vi "SetMeasureInterval.vi"(7 "SMU":T1, 8 "Error In":errorcluster, 10 "Interval":dbl, 11 "Keithley 2602 In":refnum<visa-resource-name>) -> (0 "Error Out":errorcluster, 3 "Keithley 2602 Out":refnum<visa-resource-name>)   [LabVIEW 2013, in "Keithley-2602.lvlib"]
uses:
  Keithley-2602.lvlib
  Controls/SMU.ctl
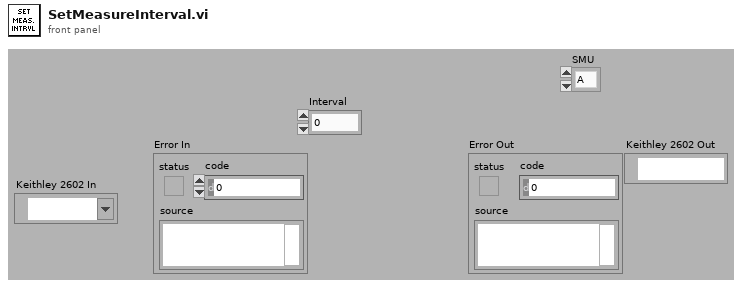
[diagram p1: front panel]
types:
  T1 = typedef "Keithley-2602.lvlib/SMU.ctl" = enum16{"A", "B"}
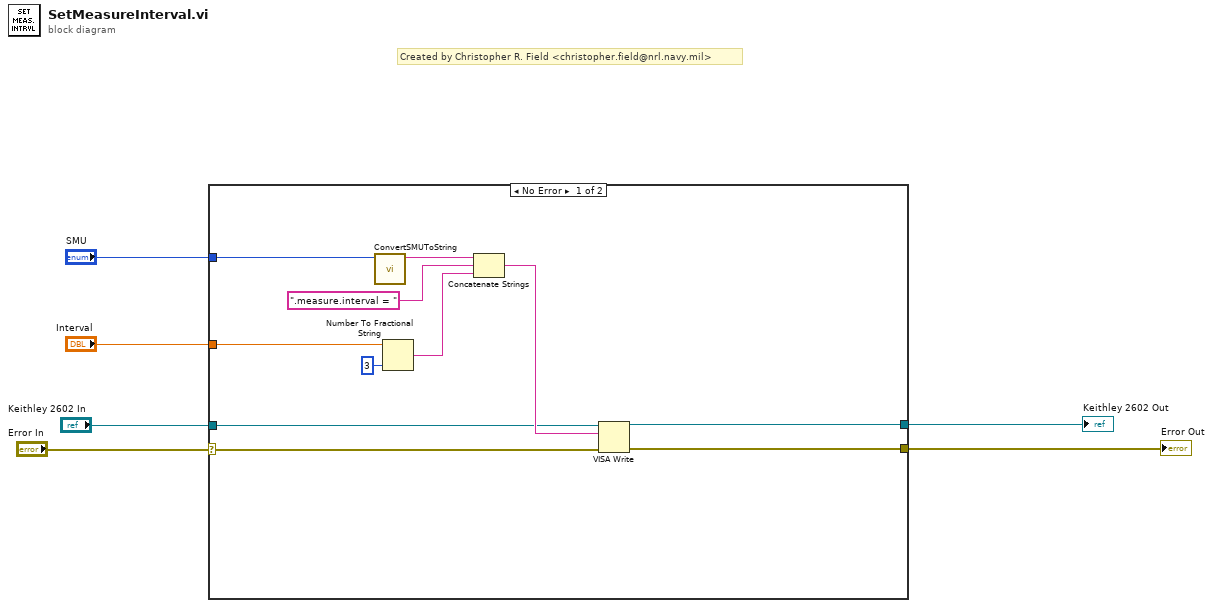
[diagram p0: block diagram]
diagram:
  # "Created by Christopher R. Field <christopher.field@nrl.navy.mil>"
  n1 = case shown="No Error" "Error In" {
    selector: "Error In" -> [w7 w18]
    tunnel: "Keithley 2602 In" -> [w14 w19]
    tunnel: [w13 w18] -> w5
    tunnel: [w12 w19] -> w4
    tunnel: "Interval" -> [w11 _]
    tunnel: "SMU" -> [w8 _]
    frame No Error {
      n2 = call "ConvertSMUToString.vi"("SMU"=w8) -> ("Channel"=w17:string)  [unwired: 10 in]
      n3 = Number To Fractional String(number=w11, precision (6)=i16 3) -> (F-format string=w9:string)  [unwired: 2 in]
      n4 = Concatenate Strings(w17, ".measure.interval = ", w9) -> (w15:string)
      n5 = VISA Write(VISA resource name=w14, write buffer=w15, error in (no error)=w7) -> (VISA resource name out=w12:refnum<visa-resource-name>, error out=w13:errorcluster)  [unwired: 1 out]
    }
    frame Error {
    }
  }
  "Error Out" <- w5
  "Keithley 2602 Out" <- w4
